vi "Panel.vi"() -> ()   [LabVIEW 2017]
panel:
  in  "Blank Button 2":bool
  in  "Blank Button":bool
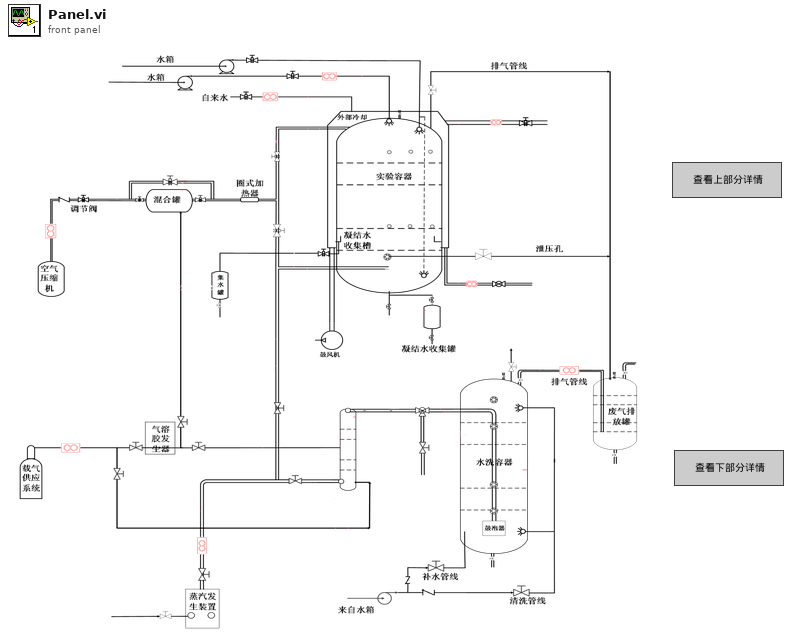
[diagram p1: front panel]
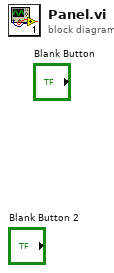
[diagram p0: block diagram]
diagram:
